vi "DANTE init & config 2.vi"(8 "Boards to configure":u8(slide) scale=0.0..8.0, 9 "DPP Configuration":T1={"reset_recovery_time"=300, "edge_peaking_time"=1, "flat_top"=6, "peaking_time"=10, "gain"=1.0, "max_risetime"=30.0, "fast_filter_thr"=25, "zero_peak_freq"=0.0, "inverted_input"=0, "base_offset"=0, "reset_threshold"=0, "overflow_recovery"=30, "tail_coefficient"=0.0, "energy_filter_thr"=25, "energy_baseline_thr"=25, "max_peaking_time"=10, "edge_flat_top"=1, "time_constant"=0.0, "baseline_samples"=0, "other_param"=0}, 10 "Number of boards in chain":u8(slide)=1 scale=1.0..8.0, 11 "IP Address":string="10.96.0.110") -> (0 "DANTE configured":bool, 1 "DANTE loaded":bool, 2 "IP added":bool, 3 "Library Initialized":bool, 5 "identifier out":string)   [LabVIEW 2015]
uses:
  XGL_DPP.lvlib
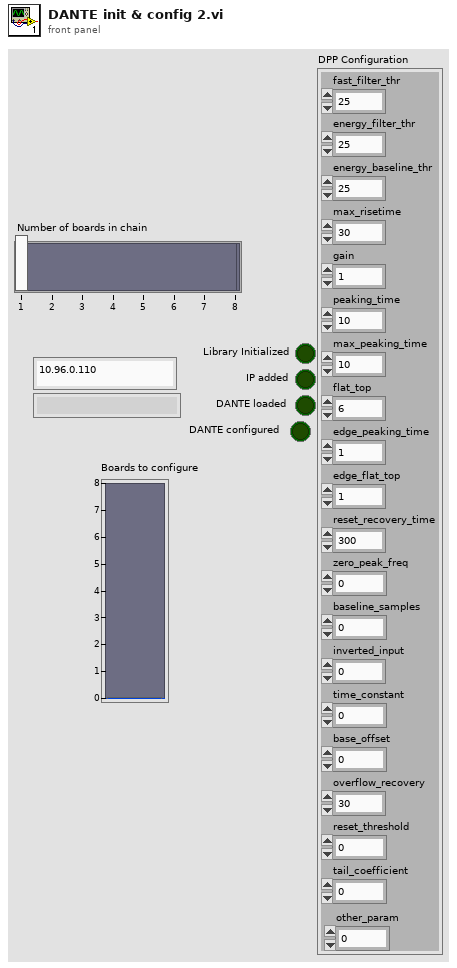
[diagram p1: front panel]
types:
  T1 = cluster{"reset_recovery_time":u32, "edge_peaking_time":u32, "flat_top":u32, "peaking_time":u32, "gain":dbl, "max_risetime":dbl, "fast_filter_thr":u32, "zero_peak_freq":dbl, "inverted_input":u8, "base_offset":u32, "reset_threshold":u32, "overflow_recovery":u32, "tail_coefficient":dbl, "energy_filter_thr":u32, "energy_baseline_thr":u32, "max_peaking_time":u32, "edge_flat_top":u32, "time_constant":dbl, "baseline_samples":u32, "other_param":u32}
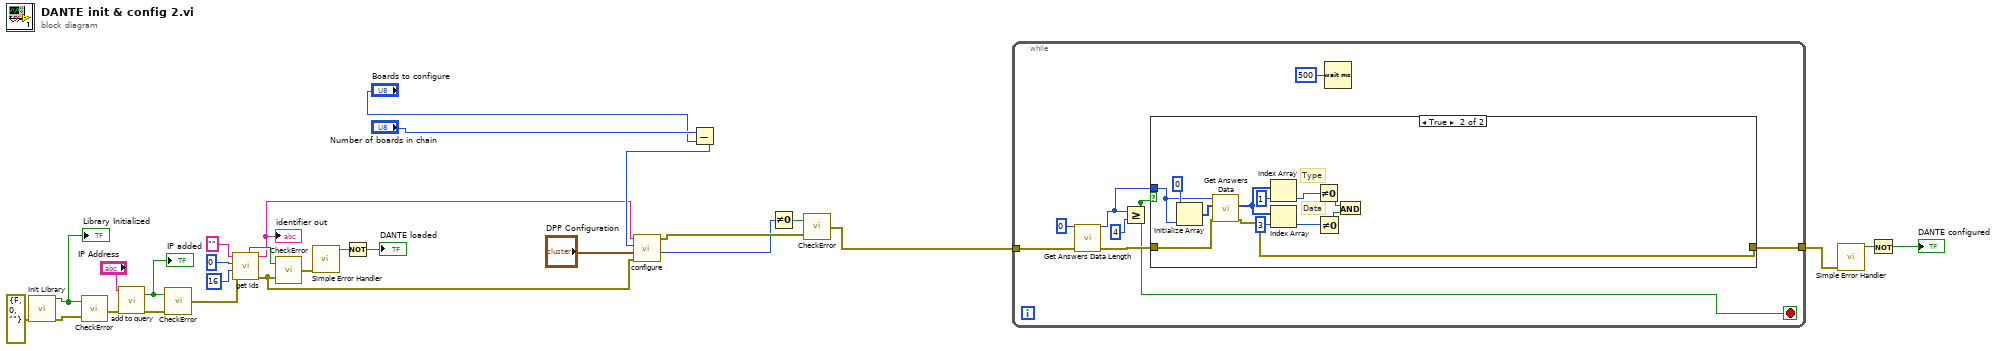
[diagram p0: block diagram]
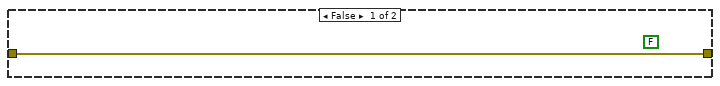
[diagram p2: hidden frame]
diagram:
  n1 = call "Init Library.vi"("error in (no error)"=errorcluster {"status"=FALSE, "code"=0, "source"=""}) -> ("error out"=w15:errorcluster, "function return"=w16:bool)  [unwired: 9 in]
  "Library Initialized" <- w16
  n2 = call "CheckError.vi"("error in (no error)"=w15, "ret_val"=w16) -> ("error out"=w17:errorcluster)
  n3 = call "add to query.vi"("error in (no error)"=w17, "address"="IP Address") -> ("error out"=w19:errorcluster, "function return"=w20:bool)  [unwired: 7 in, 1 out]
  "IP added" <- w20
  n4 = call "CheckError.vi"("error in (no error)"=w19, "ret_val"=w20) -> ("error out"=w25:errorcluster)
  n5 = call "get ids.vi"("error in (no error)"=w25, "id_size"=u32 16 ("char_size"), "nb"=u32 0, "identifier"="") -> ("error out"=w6:errorcluster, "identifier out"=w7:string, "function return"=w22:bool)  [unwired: 3 in, 2 out]
  "identifier out" <- w7
  n6 = call "CheckError.vi"("error in (no error)"=w6, "ret_val"=w22) -> ("error out"=w26:errorcluster)
  n7 = call <vilib>:"Simple Error Handler.vi"("error in (no error)"=w26) -> ("error?"=w27:bool)  [unwired: 4 in, 4 out]
  n8 = Not(x=w27) -> (.not. x?=→"DANTE loaded":bool)
  n9 = Subtract(x="Number of boards in chain", y="Boards to configure") -> (x-y=w12:u8)
  n10 = call "configure.vi"("error in (no error)"=w6, "DPP Configuration"="DPP Configuration", "Board"=w12, "identifier"=w7) -> ("function return"=w10:u32, "error out"=w11:errorcluster)  [unwired: 2 in]
  n11 = Not Equal To 0?(x=w10) -> (x != 0?=w13:bool)
  n12 = call "CheckError.vi"("error in (no error)"=w11, "ret_val"=w13) -> ("error out"=w2:errorcluster)
  n13 = while {
    tunnel: w2 -> [w32]
    tunnel: [w31] -> w1
    stop <- w29 stop-if-true
    n14 = call "Get Answers Data Length.vi"("error in (no error)"=w32, "length"=u32 0) -> ("error out"=w34:errorcluster, "length out"=w33:u32)  [unwired: 7 in, 1 out]
    n15 = Greater Or Equal?(x=w33, y=u32 4) -> (x >= y?=w29:bool)
    n16 = case shown="True" w29 {
      tunnel: w34 -> [w37 w40]
      tunnel: w33 -> [_ w42]
      tunnel: [w37 w39] -> w31
      frame False {
        (unwired) FALSE
      }
      frame True {
        # "Data"
        # "Type"
        n17 = Initialize Array(u32 0 ("y"), w42) -> (w41:u32[])
        n18 = call "Get Answers Data.vi"("error in (no error)"=w40, "data"=w41, "length"=w42) -> ("error out"=w39:errorcluster, "data out"=w38:u32[])  [unwired: 4 in, 1 out]
        n19 = Index Array(array=w38, index=1) -> (element=w45:u32)
        n20 = Index Array(array=w38, index=3) -> (element=w46:u32)
        n21 = Not Equal To 0?(x=w45) -> (x != 0?=w43:bool)
        n22 = Not Equal To 0?(x=w46) -> (x != 0?=w44:bool)
        n23 = And(x=w43, y=w44) -> ()  [unwired: 1 out]
      }
    }
    n24 = Wait (ms)(milliseconds to wait=u32 500) -> ()  [unwired: 1 out]
  }
  n25 = call <vilib>:"Simple Error Handler.vi"("error in (no error)"=w1) -> ("error?"=w3:bool)  [unwired: 4 in, 4 out]
  n26 = Not(x=w3) -> (.not. x?=→"DANTE configured":bool)
